vi "Start Command.vi"(8 "error in (no error)":errorcluster, 11 "Command in":refnum<class "Release.lvclass">) -> (0 "error out":errorcluster, 3 "Command out":refnum<class "Release.lvclass">)   [LabVIEW 2014, in "Grabber.lvlib" / "Release.lvlib" / "Release.lvclass"]
uses:
  Release.lvclass
  Robot Actor Framework/Command Actor/Command Actor Messages/FInished Command Msg/Finish Command Msg.lvclass
  <vilib>/ActorFramework/Actor/Actor.lvclass/Actor.ctl
  <vilib>/ActorFramework/Message Enqueuer/Message Enqueuer.lvclass/Message Enqueuer.ctl
  <vilib>/ActorFramework/Message Enqueuer/Init from Existing Queue.vi
  <vilib>/ActorFramework/Message Enqueuer/Enqueue.vi
  <vilib>/ActorFramework/Message Priority Queue/Priority Enqueue.vi
  <vilib>/ActorFramework/Message Enqueuer/Message Enqueuer.lvclass
  Grabber Messages/Open Arms Msg/Open Arms Msg.lvclass
  Robot Actor Framework/Command Actor/Command Actor Class/Command Actor.lvclass
  <vilib>/ActorFramework/Actor/Actor.lvclass
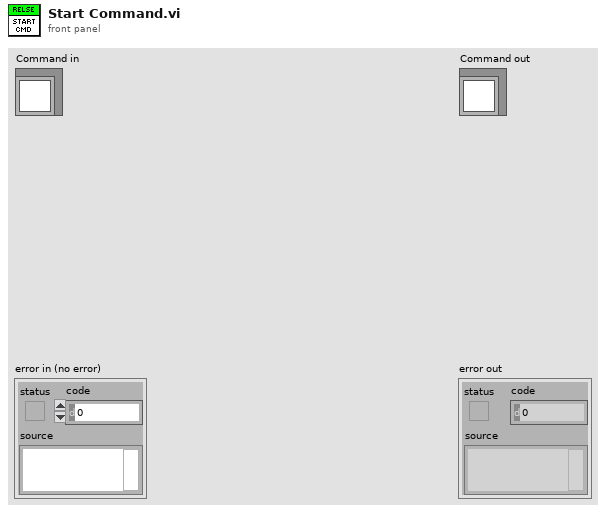
[diagram p1: front panel]
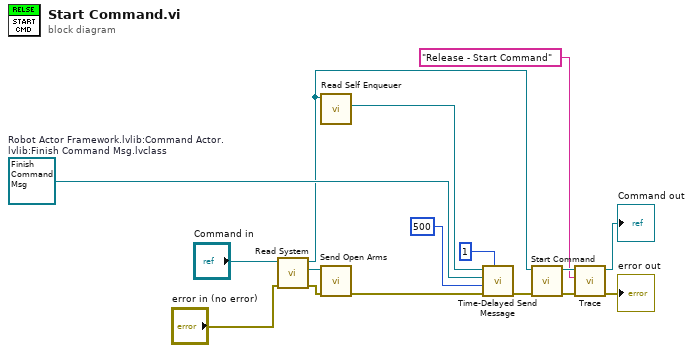
[diagram p0: block diagram]
diagram:
  w7 = refnum<class "Finish Command Msg.lvclass"> refnum  # Robot Actor Framework.lvlib:Command Actor.lvlib:Finish Command Msg.lvclass
  n1 = call-dynamic "Read System.vi"("error in (no error)"="error in (no error)", "Command in"="Command in") -> ("error out"=w10:errorcluster, "Actor Framework:Message Enqueuer"=w3:refnum<class "Message Enqueuer.lvclass">, "Command out"=w6:refnum<class "Release.lvclass">)  [unwired: 7 in]
  n2 = call <vilib>:"Read Self Enqueuer.vi"("Actor"=w6) -> ("Self Enqueuer"=w5:refnum<class "Message Enqueuer.lvclass">)  [unwired: 10 in]
  n3 = call "Send Open Arms.vi"("error in (no error)"=w10, "Message Enqueuer"=w3) -> ("error out"=w9:errorcluster)  [unwired: 8 in, 1 out]
  n4 = call <vilib>:"Time-Delayed Send Message.vi"("# Copies (0 = infinite repeat)"=u32 1, "error in (no error)"=w9, "Milliseconds To Wait"=500, "Message"=w7, "Message Enqueuer"=w5) -> ("error out"=w8:errorcluster)  [unwired: 5 in, 1 out]
  n5 = call-parent "Start Command.vi"("error in (no error)"=w8, "Command in"=w6) -> ("error out"=w13:errorcluster, "Command out"=w15:refnum<class "Release.lvclass">)  [unwired: 8 in]
  n6 = call-dynamic "Trace.vi"("error in (no error)"=w13, "Command Action"="Release - Start Command", "Command Actor in"=w15) -> ("error out"=→"error out":errorcluster, "Command Actor out"=→"Command out":refnum<class "Release.lvclass">)  [unwired: 7 in]
